vi "Motion-Poll-YAxis.vi"(8 "error in (no error)":errorcluster, 11 "Motion-ControlAll in":refnum<class "Motion-ControlAll.lvclass">) -> (0 "error out":errorcluster, 2 "Y axis \nstopped":bool, 3 "Motion-ControlAll out":refnum<class "Motion-ControlAll.lvclass">)   [LabVIEW 2013, in "Motion-ControlAll.lvclass"]
uses:
  Motion-ControlAll.lvclass
  Motion-ControlAll.lvclass/Motion-ControlAll.ctl
  <vilib>/Utility/error.llb/whitespace.ctl
  <vilib>/addons/_LabVIEW Style Book/Utilities/Style Book Utilities.lvlib
panel:
  out "Read 2":string
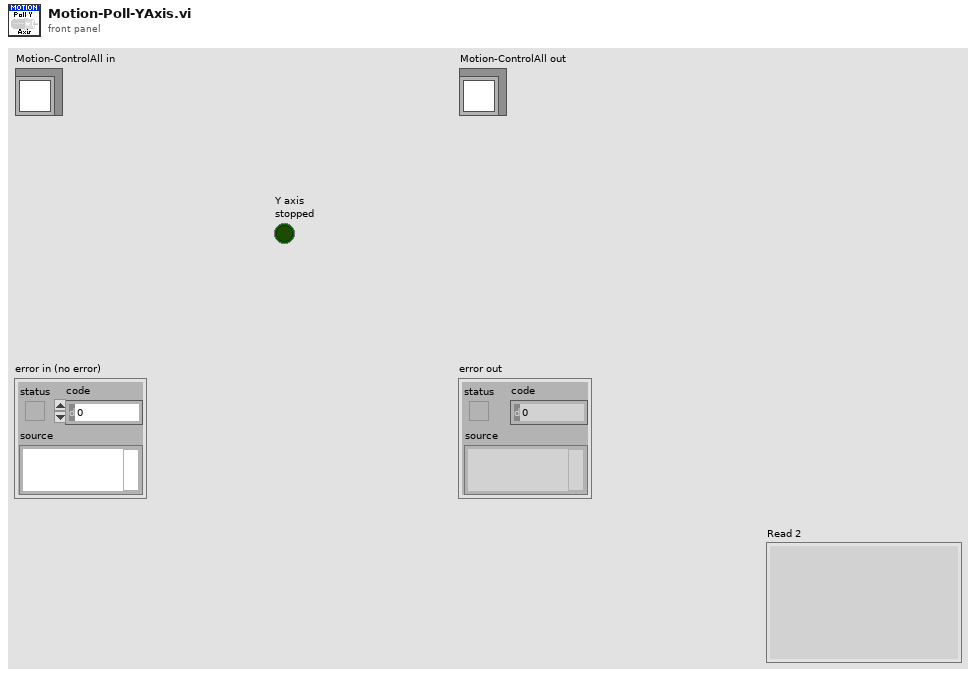
[diagram p1: front panel]
types:
  T1 = typedef "whitespace.ctl" = u16
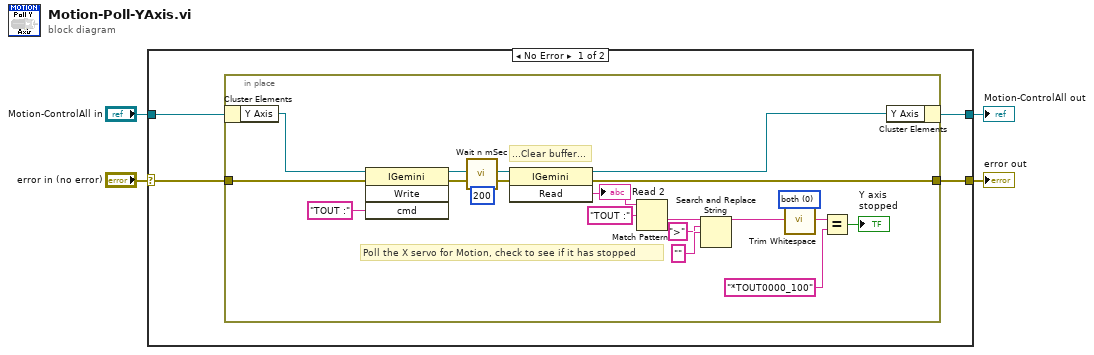
[diagram p0: block diagram]
diagram:
  n1 = case shown="No Error" "error in (no error)" {
    selector: "error in (no error)" -> [w5 w29]
    tunnel: [w7 w29] -> w3
    tunnel: [w6 w28] -> w1
    tunnel: "Motion-ControlAll in" -> [w8 w28]
    frame No Error {
      n2 = in-place {
        in-place-border: [w11] -> w7
        in-place-border: w5 -> [w9]
        w14 = T1 0 items=["both", "start of string", "end of string"] ("location (both)")
        # "Poll the X servo for Motion, check to see if it has stopped"
        # "...Clear buffer..."
        n3 = in-place-cluster #1(w8) -> ("Y Axis"=w12:refnum<k7>)
        n4 = invoke class="IGemini" method="Write"(reference=w12, error in=w9, "cmd"="TOUT :") -> (reference out=w18:refnum<k7>, error out=w19:errorcluster)  [unwired: 1 in, 2 out]
        n5 = call <vilib>:"Wait n mSec.vi"("error in (no error)"=w19, "Milliseconds to Wait (500)"=u32 200) -> ("error out"=w20:errorcluster)  [unwired: 13 in]
        n6 = invoke class="IGemini" method="Read"(reference=w18, error in=w20) -> (reference out=w10:refnum<k7>, error out=w11:errorcluster, "Read"=w17:string)  [unwired: 1 in]
        "Read 2" <- w17
        n7 = Match Pattern(string=w17, regular expression="TOUT :") -> (after substring=w23:string)  [unwired: 1 in, 3 out]
        n8 = Search and Replace String(input string=w23, search string=">", replace string="" ("replace string (\"\")")) -> (result string=w26:string)  [unwired: 5 in, 3 out]
        n9 = call <vilib>:"Trim Whitespace.vi"("string"=w26, "location (both)"=w14) -> ("trimmed string"=w13:string)
        n10 = Equal?(x=w13, y="*TOUT0000_100") -> (x = y?=→"Y axis \nstopped":bool)
        n11 = in-place-cluster #1("Y Axis"=w10) -> (w6:refnum<class "Motion-ControlAll.lvclass">)
      }
    }
    frame Error {
    }
  }
  "error out" <- w3
  "Motion-ControlAll out" <- w1
